vi "AppData_FGV.vi"(0 "Mode":enum16{"Get", "Set", "Reset"}(ring), 2 "AppData in":T1, 5 "error in (no error)":errorcluster) -> (16 "AppData out":T1, 19 "error out":errorcluster)   [LabVIEW 2019, in "Service.lvlib"]
uses:
  Service.lvlib
  AppData.ctl
  MsgQ/TypeDefs/CommandsQ.ctl
  MsgQ/TypeDefs/MsgQ_Commands.ctl
  MsgQ/MsgQ.lvlib
panel:
  # "C:\\ProgramData\\Noffz\\mmW_instr\\BH_PID.json"
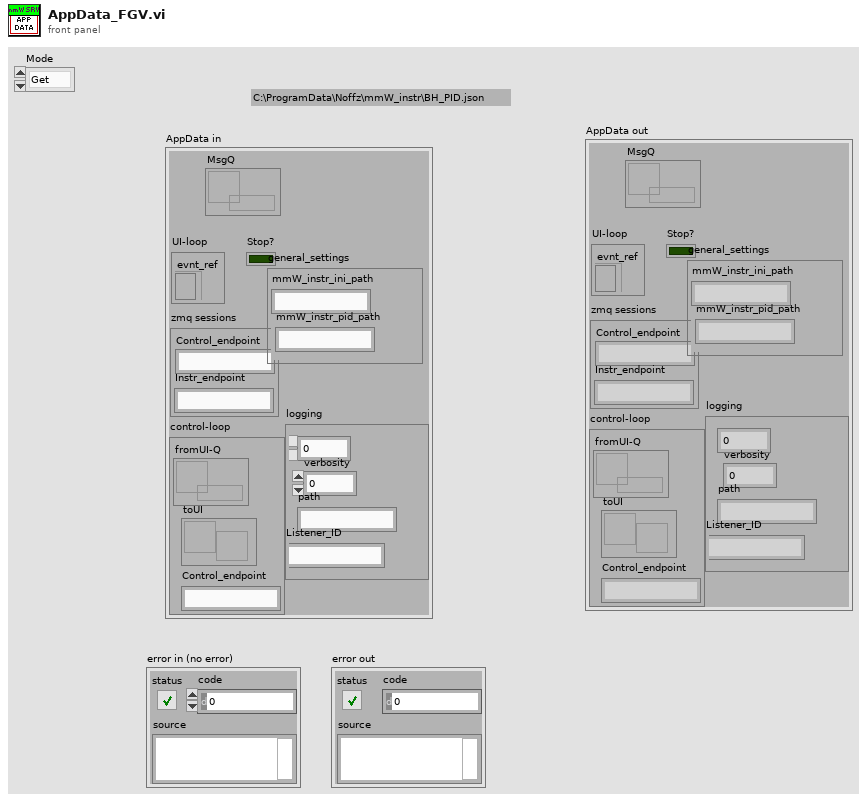
[diagram p1: front panel]
types:
  T1 = typedef "Service.lvlib/AppData.ctl" = cluster{"MsgQ":refnum<queue>, "Stop?":bool, "zmq sessions":cluster{"Control_endpoint":string, "Instr_endpoint":string}, "control-loop":cluster{"fromUI-Q":refnum<queue>, "toUI":refnum<user-event>, "Control_endpoint":string}, "UI-loop":cluster{"evnt_ref":refnum<event-registration>}, "logging":cluster{"level":dbl, "verbosity":dbl, "path":string, "Listener_ID":string}, "general_settings":cluster{"mmW_instr_ini_path":string, "mmW_instr_pid_path":string}}
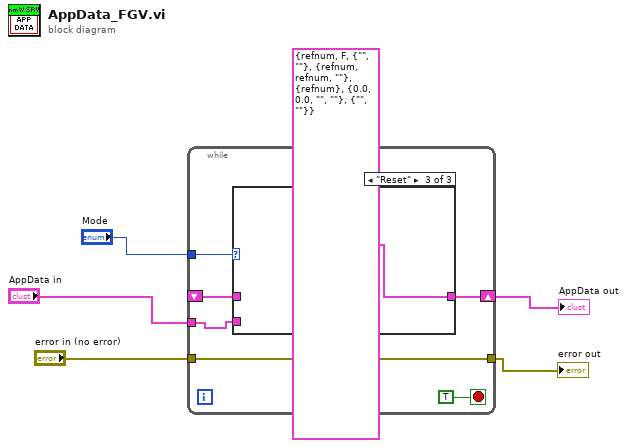
[diagram p0: block diagram]
diagram:
  n1 = while {
    tunnel: "error in (no error)" -> [w11]
    tunnel: [w11] -> w2
    tunnel: "Mode" -> [w9]
    shift-right: [w8] -> w5
    shift-left: _ -> [w7]
    tunnel: "AppData in" -> [w6]
    stop <- TRUE stop-if-true
    n2 = case shown="\"Reset\"" w9 {
      tunnel: w7 -> [w12 _ _]
      tunnel: [w12 w13 T1 {"MsgQ"=refnum, "Stop?"=FALSE, "zmq sessions"={"Control_endpoint"="", "Instr_endpoint"=""}, "control-loop"={"fromUI-Q"=refnum, "toUI"=refnum, "Control_endpoint"=""}, "UI-loop"={"evnt_ref"=refnum}, "logging"={"level"=0.0, "verbosity"=0.0, "path"="", "Listener_ID"=""}, "general_settings"={"mmW_instr_ini_path"="", "mmW_instr_pid_path"=""}}] -> w8
      tunnel: w6 -> [_ w13 _]
      frame "Get", Default {
      }
      frame "Set" {
      }
      frame "Reset" {
      }
    }
  }
  "AppData out" <- w5
  "error out" <- w2
